vi "Normalize.vi"(10 "Detrended Signal Waveform In":waveform(dbl)) -> (0 "Offset":dbl format="%0.2f", 1 "Scale":dbl format="%0.2f", 2 "Normalized Signal Waveform Out":waveform(dbl))   [LabVIEW 2025]
panel:
  out "Error Out":errorcluster
  in  "Error In":errorcluster
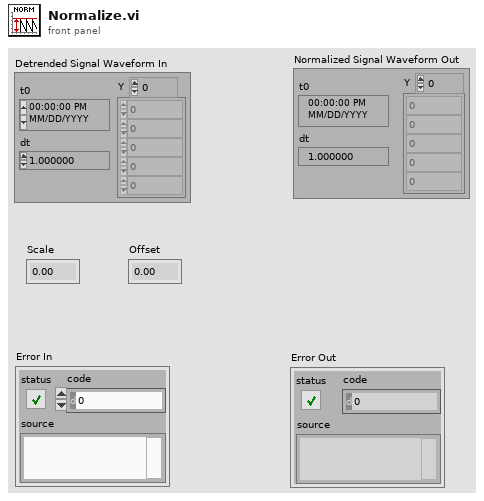
[diagram p1: front panel]
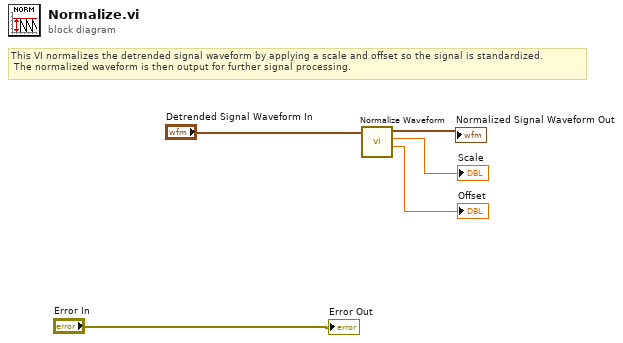
[diagram p0: block diagram]
diagram:
  # "This VI normalizes the detrended signal waveform by applying a scale and offset so the signal is standardized.\n The normalized waveform is then output for further signal processing."
  n1 = call <vilib>:"Normalize Waveform.vi"("waveform in"="Detrended Signal Waveform In") -> ("offset"=→"Offset":dbl, "scale"=→"Scale":dbl, "normalized waveform"=→"Normalized Signal Waveform Out":waveform(dbl))  [unwired: 7 in, 1 out]
  "Error Out" <- "Error In"
